vi "Configurator_Main.vi"() -> ()   [LabVIEW 2013]
doc: "This is the main VI for the configuration editor."
uses:
  Controls/StateCluster.ctl
  vi.lib/CEF_TreeControl/Repository/NISE_CEF_Repository.lvclass
  vi.lib/CEF_TreeControl/Node/NodeRef.ctl
  vi.lib/CEF_TreeControl/Node/NISE_CEF_Node.lvclass
  vi.lib/CEF_TreeControl/Node/UserEventRef.ctl
  vi.lib/CEF_TreeControl/Controls/EventCluster.ctl
  Controls/AddMessage.ctl
  Controls/MoveMessage.ctl
  Classes/cRIO/cRIO.lvclass
  Classes/cRIO Repo/cRIORepo.lvclass
  <vilib>/NI/AMC/Read Termination Message.vi
  <vilib>/NI/AMC/Create Single Message.vi
  <vilib>/NI/AMC/Update Message Routing Info.vi
  <vilib>/NI/AMC/Send Message.vi
  <vilib>/NI/AMC/Globals.vi
  <vilib>/NI/AMC/AMC.lvlib
  vi.lib/CEF_TreeControl/NISE_CEF_TreeControl.lvlib
panel:
  in  "View":string(tree)
  in  "Exit":bool
  # "Configurator"
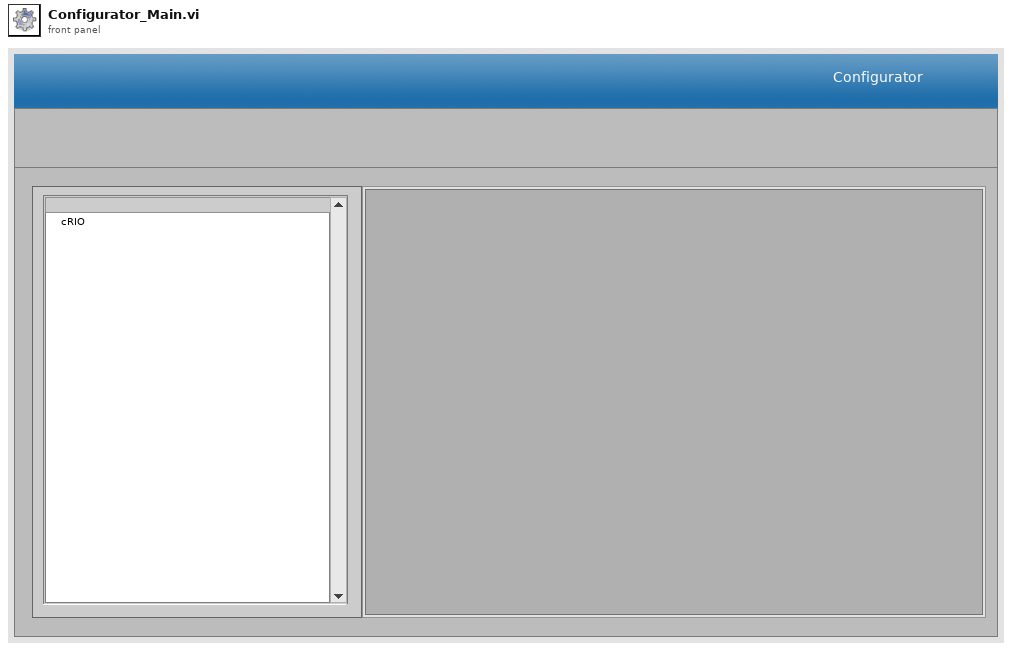
[diagram p1: front panel]
types:
  T1 = typedef "StateCluster.ctl" = cluster{"repository":refnum<class "NISE_CEF_Repository.lvclass">, "root":T2, "unsaved changes":bool, "current path":path, "user event ref":T3, "glyph path":path, "classes path":path}
  T2 = typedef "NISE_CEF_Node.lvclass/NodeRef.ctl" = refnum<data-value>
  T3 = typedef "NISE_CEF_Node.lvclass/UserEventRef.ctl" = refnum<user-event>
  T4 = typedef "AMC.lvlib/Message Queue.ctl" = refnum<queue>
  T5 = typedef "AddMessage.ctl" = cluster{"node type":string, "to add to":string}
  T6 = typedef "MoveMessage.ctl" = cluster{"node ref":T2, "new parent":T2}
  T7 = typedef "NISE_CEF_TreeControl.lvlib/EventCluster.ctl" = cluster{"command":string, "data":string}
  T8 = typedef "FilePaths.ctl" = cluster{"glyphs":path, "classes":path}
  T9 = typedef "NISE_CEF_Node.lvclass/Summary.ctl" = cluster{"ID":string, "parent ID":string, "node type":string, "text":string, "additional text":string, "glyph":string, "depth":i32}
  T10 = typedef "LVPoint32TypeDef.ctl" = cluster{"Horizontal":i32, "Vertical":i32}
  T11 = cluster{"data name":string, "drag data":variant}[]
  T12 = typedef "NISE_CEF_Node.lvclass/NodeMenuOptions.ctl" = cluster{"removable":bool, "movable":bool, "duplicate":bool}
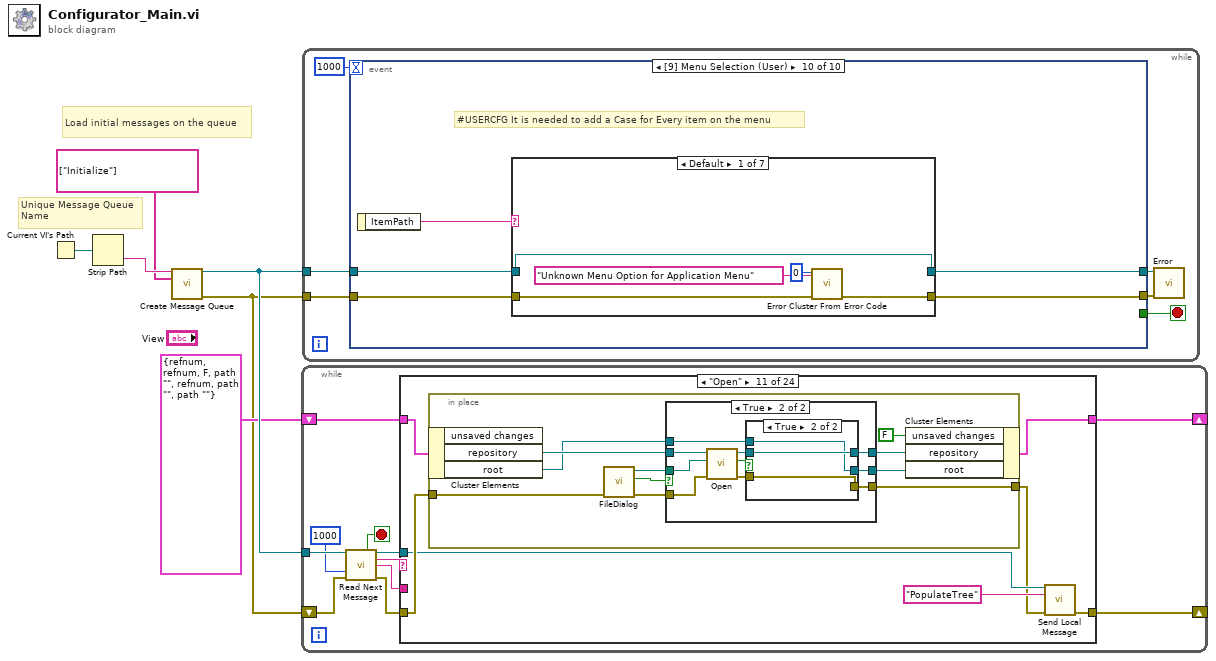
[diagram p0: block diagram]
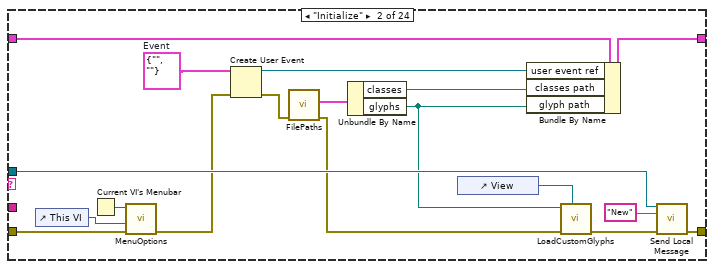
[diagram p3: hidden frame]
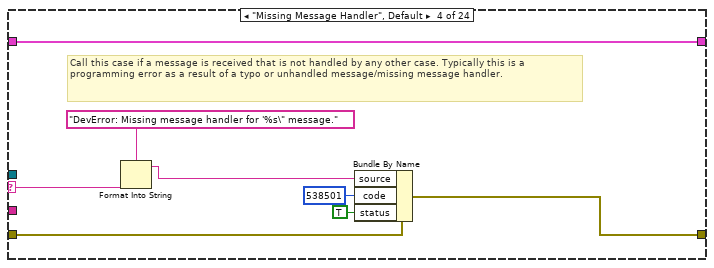
[diagram p5: hidden frame]
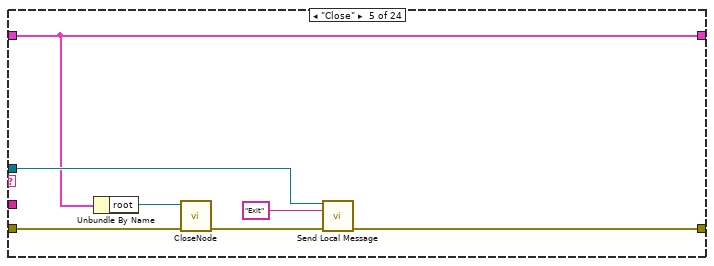
[diagram p6: hidden frame]
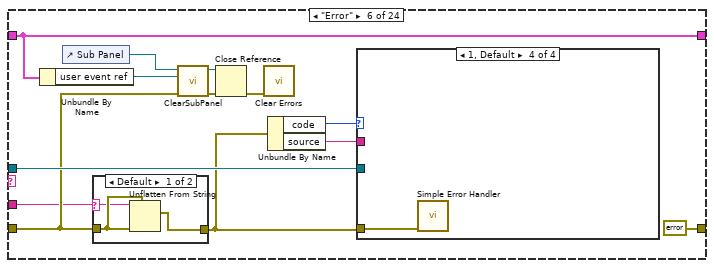
[diagram p7: hidden frame]
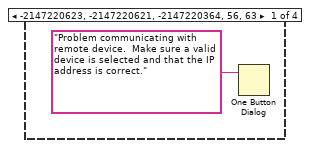
[diagram p9: hidden frame]
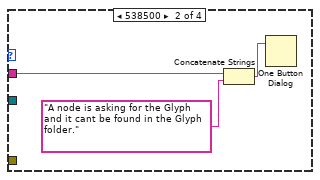
[diagram p10: hidden frame]
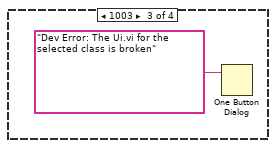
[diagram p11: hidden frame]
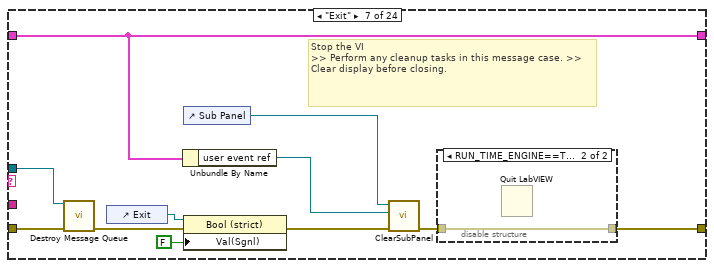
[diagram p12: hidden frame]
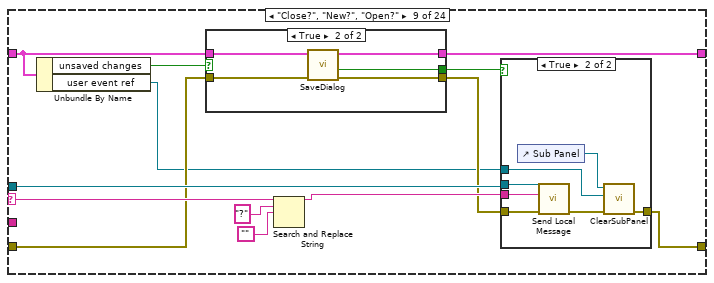
[diagram p15: hidden frame]
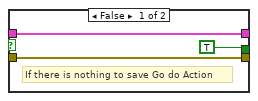
[diagram p16: hidden frame]
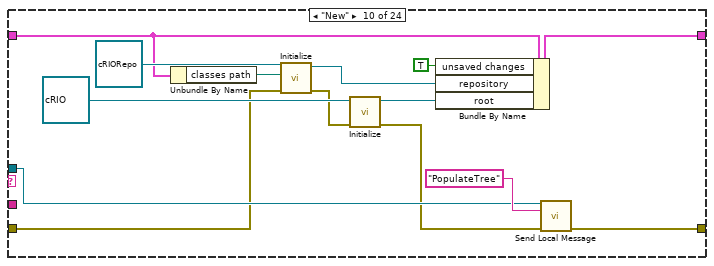
[diagram p18: hidden frame]
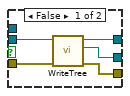
[diagram p20: hidden frame]
diagram:
  # "Unique Message Queue Name"
  # "Load initial messages on the queue"
  n1 = Current VI's Path() -> (path=w5:path)
  n2 = Strip Path(path=w5) -> (name=w6:string)  [unwired: 1 out]
  n3 = call <vilib>:"Create Message Queue.vi"("message queue name"=w6, "initial message names"=string[] ["Initialize"]) -> ("message queue out"=w3:T4, "error out"=w1:errorcluster)  [unwired: 12 in]
  n4 = while "Message Processor" {
    shift-right: [w13] -> _
    shift-left: w1 -> [w12]
    tunnel: w3 -> [w11]
    shift-right: [w9] -> _
    shift-left: T1 {"repository"=refnum, "root"=refnum, "unsaved changes"=FALSE, "current path"=path "", "user event ref"=refnum, "glyph path"=path "", "classes path"=path ""} -> [w8]
    stop <- w17 stop-if-true
    n5 = call <vilib>:"Read Next Message.vi"("message queue in"=w11, "timeout (1 ms)"=1000, "error in"=w12) -> ("exit process?"=w17:bool, "message queue out"=w7:T4, "message name"=w16:string, "message value"=w15:string, "error out"=w14:errorcluster)  [unwired: 5 in, 3 out]
    n6 = case shown="\"Open\"" w16 {
      selector: w16 -> [_ _ _ w46 _ _ _ _ w101 _ _ _ _ _ _ _ _ w277 _ _ _ _ _ _]
      tunnel: w15 -> [_ _ _ _ _ w56 _ _ _ _ _ _ _ w210 _ w247 w258 w275 w311 w332 _ _ w368 w388]
      tunnel: w14 -> [w19 w37 w39 w44 w49 w59 w88 w92 w94 w122 w140 w176 w202 w217 w230 w236 w257 w280 w313 w331 w348 w358 w367 w386]
      tunnel: [w19 w31 w39 w43 w53 errorcluster {"status"=FALSE, "code"=0, "source"=""} ("error out") w80 w92 w105 w134 w136 w180 w204 w214 w230 w239 w261 w283 w317 w328 w342 w353 w364 w381] -> w13
      tunnel: [w18 w26 w38 w45 w51 w64 w79 w91 w96 w132 w141 w183 w203 w211 w229 w233 w262 w284 w315 w333 w352 w357 w362 w389] -> w9
      tunnel: w8 -> [w18 w27 w38 w45 w51 w64 w79 w91 w97 w126 w142 w178 w201 w212 w229 w234 w262 w284 w316 w333 w352 w357 w362 w389]
      tunnel: w7 -> [_ w30 _ _ w52 w67 w87 _ w104 w133 w138 w179 _ w213 _ _ _ w278 _ _ _ _ w363 w380]
      frame "------------Generic Operations------------" {
        # "Dummy case to add a seperation in the Case Structure menu"
      }
      frame "Initialize" {
        w21 = T7 {"command"="", "data"=""}  # Event
        n7 = control-ref of="This VI"() -> (w36:refnum<vi>)
        n8 = Current VI's Menubar() -> (w35:refnum<k9>)
        n9 = call "MenuOptions.vi"("error in"=w37, "VI ref"=w36, "menu ref in"=w35) -> ("error out"=w25:errorcluster)  [unwired: 7 in, 1 out]
        n10 = Create User Event(user event datatype=w21, error in=w25) -> (user event=w20:refnum<user-event>, error out=w24:errorcluster)
        n11 = call "FilePaths.vi"("error in"=w24) -> ("error out"=w29:errorcluster, "paths"=w28:T8)  [unwired: 9 in]
        n12 = Unbundle By Name(w28) -> ("classes"=w23:path, "glyphs"=w22:path)
        n13 = control-ref of="View"() -> (w34:refnum<vi>)
        n14 = Bundle By Name(cluster=w27, "user event ref"=w20, "classes path"=w23, "glyph path"=w22) -> (w26:T1)
        n15 = call "LoadCustomGlyphs.vi"("tree ref"=w34, "error in"=w29, "glyph directory"=w22) -> ("error out"=w32:errorcluster)  [unwired: 8 in]
        n16 = call <vilib>:"Send Local Message.vi"("message queue in"=w30, "message name"="New" ("Message Name"), "error in"=w32) -> ("error out"=w31:errorcluster)  [unwired: 10 in, 2 out]
      }
      frame "", "Idle" {
      }
      frame "Missing Message Handler", Default {
        # "Call this case if a message is received that is not handled by any other case. Typically this is a programming error as a result of a typo or unhandled message/missing message handler."
        n17 = Format Into String(format string="DevError: Missing message handler for '%s\" message." ("message"), w46) -> (resulting string=w40:string)  [unwired: 2 in, 1 out]
        n18 = Bundle By Name(cluster=w44, "source"=w40, "code"=538501, "status"=TRUE) -> (w43:errorcluster)
      }
      frame "Close" {
        n19 = Unbundle By Name(w51) -> ("root"=w50:T2)
        n20 = call "CloseNode.vi"("error in"=w49, "node ref"=w50) -> ("error out"=w48:errorcluster)  [unwired: 9 in]
        n21 = call <vilib>:"Send Local Message.vi"("message queue in"=w52, "message name"="Exit", "error in"=w48) -> ("error out"=w53:errorcluster)  [unwired: 10 in, 2 out]
      }
      frame "Error" {
        n22 = Unbundle By Name(w64) -> ("user event ref"=w62:T3)
        n23 = control-ref of="Sub Panel"() -> (w63:refnum<vi>)
        n24 = case shown="Default" w56 {
          selector: w56 -> [w69 _]
          tunnel: w59 -> [w70 w71]
          tunnel: [w68 w71] -> w58
          frame Default {
            n25 = Unflatten From String(type=w70, binary string=w69, error in (no error)=w70) -> (value=w68:errorcluster)  [unwired: 2 in, 2 out]
          }
          frame "" {
          }
        }
        n26 = call "ClearSubPanel.vi"("error in"=w59, "user event ref"=w62, "sub panel ref in"=w63) -> ("error out"=w61:errorcluster, "sub panel ref out"=w60:refnum<vi>)  [unwired: 7 in]
        n27 = Close Reference(reference=w60, error in (no error)=w61) -> (error out=w57:errorcluster)
        n28 = call <vilib>:"Clear Errors.vi"("error in (no error)"=w57) -> ()  [unwired: 6 in, 1 out]
        n29 = Unbundle By Name(w58) -> ("code"=w65:i32, "source"=w55:string)
        n30 = case shown="1, Default" w65 {
          tunnel: w67 -> [_ _ _ _]
          tunnel: w58 -> [_ _ _ w77]
          tunnel: w55 -> [_ w75 _ _]
          frame -2147220623, -2147220621, -2147220364, 56, 63 {
            n31 = One Button Dialog(message="Problem communicating with remote device.  Make sure a valid device is selected and that the IP address is correct.") -> ()  [unwired: 1 in, 1 out]
          }
          frame 538500 {
            n32 = Concatenate Strings(w75, "A node is asking for the Glyph and it cant be found in the Glyph folder." ("message")) -> (w73:string)
            n33 = One Button Dialog(message=w73) -> ()  [unwired: 1 in, 1 out]
          }
          frame 1003 {
            n34 = One Button Dialog(message="Dev Error: The Ui.vi for the selected class is broken") -> ()  [unwired: 1 in, 1 out]
          }
          frame 1, Default {
            n35 = call <vilib>:"Simple Error Handler.vi"("error in (no error)"=w77) -> ()  [unwired: 1 in, 8 out]
          }
        }
      }
      frame "Exit" {
        # "Stop the VI                                                                             >> Perform any cleanup tasks in this message case. >> Clear display before closing."
        n36 = call <vilib>:"Destroy Message Queue.vi"("message queue in"=w87, "error in"=w88) -> ("error out"=w84:errorcluster)  [unwired: 11 in, 2 out]
        n37 = control-ref of="Exit"() -> (w86:refnum<vi>)
        n38 = Unbundle By Name(w79) -> ("user event ref"=w78:T3)
        n39 = control-ref of="Sub Panel"() -> (w83:refnum<vi>)
        n40 = property class="Bool (strict)"(reference=w86, error in=w84, "Val(Sgnl)"=FALSE ("Exit")) -> (error out=w82:errorcluster)  [unwired: 1 out]
        n41 = call "ClearSubPanel.vi"("error in"=w82, "user event ref"=w78, "sub panel ref in"=w83) -> ("error out"=w81:errorcluster)  [unwired: 7 in, 1 out]
        n42 = disable-structure shown="RUN_TIME_ENGINE==True" {
          disable-tunnel: [w89 w90] -> w80
          disable-tunnel: w81 -> [w89 w90]
          frame condition #0 (active) {
          }
          frame condition #1 {
            n43 = Quit LabVIEW() -> ()  [unwired: 1 in]
          }
        }
      }
      frame "------------Menu Operations--------------" {
        # "Dummy case to add a seperation in the Case Structure menu"
      }
      frame "Close?", "New?", "Open?" {
        n44 = Unbundle By Name(w97) -> ("unsaved changes"=w99:bool, "user event ref"=w93:T3)
        n45 = case shown="True" w99 {
          tunnel: [TRUE ("SaveFlag") w113] -> w98
          tunnel: w97 -> [w107 w112]
          tunnel: [w107 w111] -> w96
          tunnel: w94 -> [w106 w110]
          tunnel: [w106 w109] -> w95
          frame False {
            # "If there is nothing to save Go do Action"
          }
          frame True {
            n46 = call "SaveDialog.vi"("error in"=w110, "state in"=w112) -> ("error out"=w109:errorcluster, "new"=w113:bool, "state out"=w111:T1)  [unwired: 7 in]
          }
        }
        n47 = Search and Replace String(input string=w101, search string="?", replace string="") -> (result string=w100:string)  [unwired: 5 in, 3 out]
        n48 = case shown="True" w98 {
          tunnel: w95 -> [w114 w121]
          tunnel: [w114 w117] -> w105
          tunnel: w104 -> [_ w120]
          tunnel: w100 -> [_ w119]
          tunnel: w93 -> [_ w116]
          frame False {
          }
          frame True {
            n49 = control-ref of="Sub Panel"() -> (w115:refnum<vi>)
            n50 = call <vilib>:"Send Local Message.vi"("message queue in"=w120, "message name"=w119, "error in"=w121) -> ("error out"=w118:errorcluster)  [unwired: 10 in, 2 out]
            n51 = call "ClearSubPanel.vi"("error in"=w118, "user event ref"=w116, "sub panel ref in"=w115) -> ("error out"=w117:errorcluster)  [unwired: 7 in, 1 out]
          }
        }
      }
      frame "New" {
        n52 = Unbundle By Name(w126) -> ("classes path"=w125:path)
        n53 = call-dynamic "Initialize.vi"("error in"=w122, "path"=w125, "repository in"=refnum<class "cRIORepo.lvclass"> refnum ("cRIORepo.lvclass")) -> ("error out"=w124:errorcluster, "repository out"=w127:refnum<class "cRIORepo.lvclass">)  [unwired: 7 in]
        n54 = call-dynamic "Initialize.vi"("error in"=w124, "cRIO in"=refnum<class "cRIO.lvclass"> refnum ("cRIO.lvclass")) -> ("error out"=w123:errorcluster, "data value reference"=w129:T2)  [unwired: 7 in, 1 out]
        n55 = Bundle By Name(cluster=w126, "unsaved changes"=TRUE ("SaveFlag"), "repository"=w127, "root"=w129) -> (w132:T1)
        n56 = call <vilib>:"Send Local Message.vi"("message queue in"=w133, "message name"="PopulateTree", "error in"=w123) -> ("error out"=w134:errorcluster)  [unwired: 10 in, 2 out]
      }
      frame "Open" {
        n57 = in-place {
          in-place-border: w140 -> [w143]
          in-place-border: [w149] -> w137
          n58 = in-place-cluster #1(w142) -> ("repository"=w152:refnum<class "NISE_CEF_Repository.lvclass">, "root"=w147:T2)  [unwired: 1 out]
          n59 = call "FileDialog.vi"("error in"=w143) -> ("error out"=w144:errorcluster, "Valid"=w146:bool, "selected path"=w145:path)  [unwired: 7 in, 1 out]
          n60 = case shown="True" w146 {
            tunnel: w152 -> [w153 w165]
            tunnel: [w153 w163] -> w150
            tunnel: [w154 w161] -> w149
            tunnel: [w155 w160] -> w148
            tunnel: w145 -> [_ w158]
            tunnel: w144 -> [w154 w157]
            tunnel: w147 -> [w155 w156]
            frame False {
            }
            frame True {
              n61 = call-dynamic "Open.vi"("error in"=w157, "file path"=w158, "repository in"=w165) -> ("error out"=w162:errorcluster, "invalid?"=w159:bool, "repository out"=w164:refnum<class "NISE_CEF_Repository.lvclass">)  [unwired: 6 in]
              n62 = case shown="True" w159 {
                tunnel: w164 -> [w170 w173]
                tunnel: [w169 w173] -> w163
                tunnel: w162 -> [w168 w172]
                tunnel: [w167 w172] -> w161
                tunnel: [w166 w171] -> w160
                tunnel: w156 -> [_ w171]
                frame False {
                  n63 = call-dynamic "WriteTree.vi"("error in"=w168, "repository in"=w170) -> ("error out"=w167:errorcluster, "root"=w166:T2, "repository out"=w169:refnum<class "NISE_CEF_Repository.lvclass">)  [unwired: 7 in]
                }
                frame True {
                }
              }
            }
          }
          n64 = in-place-cluster #1("unsaved changes"=FALSE ("SaveFlag"), "repository"=w150, "root"=w148) -> (w141:T1)
        }
        n65 = call <vilib>:"Send Local Message.vi"("message queue in"=w138, "message name"="PopulateTree", "error in"=w137) -> ("error out"=w136:errorcluster)  [unwired: 10 in, 2 out]
      }
      frame "Save" {
        n66 = in-place {
          in-place-border: w176 -> [w187]
          in-place-border: [w186] -> w175
          in-place-border: [w184] -> w174
          n67 = in-place-cluster #2(w178) -> ("current path"=w185:path, "root"=w188:T2, "repository"=w190:refnum<class "NISE_CEF_Repository.lvclass">)
          n68 = Empty String/Path?(string/path=w185) -> (empty?=w184:bool)
          n69 = call-dynamic "ReadTree.vi"("error in"=w187, "root"=w188, "repository in"=w190) -> ("error out"=w186:errorcluster, "repository out"=w189:refnum<class "NISE_CEF_Repository.lvclass">)  [unwired: 7 in]
          n70 = in-place-cluster #2("current path"=w185, "root"=w188, "repository"=w189) -> (w177:T1)
        }
        n71 = case shown="True" w174 {
          tunnel: w177 -> [w194 w196]
          tunnel: [w193 w195] -> w183
          tunnel: [w192 w197] -> w181
          tunnel: w175 -> [w191 w198]
          frame False {
            n72 = call "Save.vi"("error in"=w191, "state in"=w194) -> ("error out"=w192:errorcluster, "state out"=w193:T1)  [unwired: 8 in]
          }
          frame True {
            # "Empty path use Dialog"
            n73 = call "SaveAs.vi"("error in"=w198, "state in"=w196) -> ("error out"=w197:errorcluster, "state out"=w195:T1)  [unwired: 7 in, 1 out]
          }
        }
        n74 = call <vilib>:"Send Local Message.vi"("message queue in"=w179, "message name"="PopulateTree", "error in"=w181) -> ("error out"=w180:errorcluster)  [unwired: 10 in, 2 out]
      }
      frame "SaveAs" {
        n75 = in-place {
          in-place-border: w202 -> [w206]
          in-place-border: [w205] -> w200
          n76 = in-place-cluster #3(w201) -> ("root"=w207:T2, "repository"=w209:refnum<class "NISE_CEF_Repository.lvclass">)
          n77 = call-dynamic "ReadTree.vi"("error in"=w206, "root"=w207, "repository in"=w209) -> ("error out"=w205:errorcluster, "repository out"=w208:refnum<class "NISE_CEF_Repository.lvclass">)  [unwired: 7 in]
          n78 = in-place-cluster #3("root"=w207, "repository"=w208) -> (w199:T1)
        }
        n79 = call "SaveAs.vi"("error in"=w200, "state in"=w199) -> ("error out"=w204:errorcluster, "state out"=w203:T1)  [unwired: 7 in, 1 out]
      }
      frame "Custom View" {
        n80 = in-place {
          in-place-border: w217 -> [w228]
          in-place-border: [w227] -> w215
          in-place-border: w210 -> [w218]
          n81 = in-place-cluster #4(w212) -> ("repository"=w222:refnum<class "NISE_CEF_Repository.lvclass">, "root"=w221:T2)
          n82 = call-dynamic "ReadTree.vi"("error in"=w228, "root"=w221, "repository in"=w222) -> ("error out"=w225:errorcluster, "repository out"=w224:refnum<class "NISE_CEF_Repository.lvclass">)  [unwired: 7 in]
          n83 = call-dynamic "CustomView.vi"("error in"=w225, "view name"=w218, "repository in"=w224) -> ("error out"=w226:errorcluster, "repository out"=w223:refnum<class "NISE_CEF_Repository.lvclass">)  [unwired: 7 in]
          n84 = call-dynamic "WriteTree.vi"("error in"=w226, "repository in"=w223) -> ("error out"=w227:errorcluster, "root"=w219:T2, "repository out"=w220:refnum<class "NISE_CEF_Repository.lvclass">)  [unwired: 7 in]
          n85 = in-place-cluster #4("repository"=w220, "root"=w219) -> (w211:T1)
        }
        n86 = call <vilib>:"Send Local Message.vi"("message queue in"=w213, "message name"="PopulateTree", "error in"=w215) -> ("error out"=w214:errorcluster)  [unwired: 10 in, 2 out]
      }
      frame "-------TreeControl Operations-----------" {
        # "Dummy case to add a seperation in the Case Structure menu"
      }
      frame "AddNode" {
        n87 = Unflatten From String(type=T5 {"node type"="", "to add to"=""} ("input cluster"), binary string=w247) -> (value=w245:T5)  [unwired: 3 in, 2 out]
        n88 = Unbundle By Name(w245) -> ("to add to"=w242:string, "node type"=w232:string)
        n89 = in-place {
          in-place-border: w236 -> [w253]
          in-place-border: [w252] -> w235
          in-place-border: w232 -> [w251]
          in-place-border: [w250] -> w231
          n90 = in-place-cluster #5(w234) -> ("repository"=w255:refnum<class "NISE_CEF_Repository.lvclass">)
          n91 = call-dynamic "GetClassPath.vi"("error in"=w253, "class name"=w251, "Repository in"=w255) -> ("error out"=w252:errorcluster, "class path"=w250:path, "Repository out"=w254:refnum<class "NISE_CEF_Repository.lvclass">)  [unwired: 6 in]
          n92 = in-place-cluster #5("repository"=w254) -> (w233:T1)
        }
        n93 = control-ref of="View"() -> (w237:refnum<vi>)
        n94 = call <vilib>:"Get LV Class Default Value.vi"("error in (no error)"=w235, "class path"=w231) -> ("error out"=w248:errorcluster, "object"=w249:refnum<class>)  [unwired: 8 in]
        n95 = To More Specific Class(target class=refnum<class "NISE_CEF_Node.lvclass"> refnum ("Node.lvclass"), reference=w249, error in=w248) -> (specific class reference=w244:refnum<class "NISE_CEF_Node.lvclass">, error out=w241:errorcluster)
        n96 = call "AddNode.vi"("error in"=w241, "node in"=w244, "parent node ID"=w242) -> ("error out"=w240:errorcluster, "summary"=w238:T9[])  [unwired: 7 in]
        n97 = call "PopulateTreeSumary.vi"("error in"=w240, "array"=w238, "tree ref in"=w237) -> ("error out"=w239:errorcluster)  [unwired: 8 in]
      }
      frame "Duplicate" {
        n98 = call "IDtoNode.vi"("error in"=w257, "ID"=w258) -> ("error out"=w259:errorcluster, "invalid Id"=w256:bool, "node ref"=w260:T2)  [unwired: 7 in]
        n99 = case shown="False" w256 {
          tunnel: [w271 w272] -> w261
          tunnel: w260 -> [w269 _]
          tunnel: w259 -> [w266 w272]
          frame False {
            n100 = call "DuplicateNode.vi"("same parent?"=TRUE ("s"), "error in"=w266, "node ref in"=w269) -> ("error out"=w267:errorcluster, "new node ref"=w268:T2)  [unwired: 7 in]
            n101 = call "Summary.vi"("error in"=w267, "node self ref"=w268) -> ("error out"=w264:errorcluster, "summary"=w263:T9[])  [unwired: 8 in]
            n102 = control-ref of="View"() -> (w270:refnum<vi>)
            n103 = call "PopulateTreeSumary.vi"("error in"=w264, "array"=w263, "tree ref in"=w270) -> ("error out"=w271:errorcluster)  [unwired: 8 in]
          }
          frame True {
          }
        }
      }
      frame "CustomMenuAction" {
        n104 = Match Pattern(string=w275, regular expression=":") -> (before substring=w274:string, after substring=w273:string)  [unwired: 1 in, 2 out]
        n105 = call "IDtoNode.vi"("error in"=w280, "ID"=w273) -> ("error out"=w281:errorcluster, "invalid Id"=w279:bool, "node ref"=w282:T2)  [unwired: 7 in]
        n106 = case shown="False" w279 {
          tunnel: [w285 w308] -> w283
          tunnel: w282 -> [w292 _]
          tunnel: w281 -> [w289 w308]
          tunnel: w278 -> [w291 _]
          tunnel: w277 -> [_ _]
          tunnel: w274 -> [w287 _]
          frame False {
            n107 = control-ref of="View"() -> (w290:refnum<vi>)
            n108 = in-place {
              in-place-border: w291 -> [w306]
              in-place-border: w290 -> [w304]
              in-place-border: w289 -> [w303]
              in-place-border: [w302] -> w286
              in-place-border: [w301] -> w288
              in-place-border: w287 -> [w300]
              n109 = in-place-dvr #6(w292) -> (w307:refnum<class "NISE_CEF_Node.lvclass">)  [unwired: 1 out]
              n110 = call-dynamic "MenuHandler.vi"("tree control"=w304, "message queue out"=w306, "error in (no error)"=w303, "menu string"=w300, "NISE_CEF_Node in"=w307) -> ("error out"=w302:errorcluster, "Unhandled"=w301:bool, "NISE_CEF_Node out"=w305:refnum<class "NISE_CEF_Node.lvclass">)  [unwired: 4 in]
              n111 = in-place-dvr #6(w305) -> ()  [unwired: 2 out]
            }
            n112 = case shown="True" w288 {
              tunnel: w287 -> [_ w298]
              tunnel: w286 -> [w293 w297]
              tunnel: [w293 w296] -> w285
              frame False {
              }
              frame True {
                # "Generates Error"
                n113 = Concatenate Strings("Unknown Menu item command:  " ("message"), w298) -> (w295:string)
                n114 = call <vilib>:"Error Cluster From Error Code.vi"("error in (no error)"=w297, "error message (\"\")"=w295, "error code (0)"=538502) -> ("error out"=w296:errorcluster)  [unwired: 6 in]
              }
            }
          }
          frame True {
          }
        }
      }
      frame "RefreshNode" {
        # "Refreshes the node in the Tree               Sets the save flag to true                       This case can be called from the UIs of the nodes"
        n115 = call "IDtoNode.vi"("error in"=w313, "ID"=w311) -> ("error out"=w312:errorcluster, "invalid Id"=w309:bool, "node ref"=w310:T2)  [unwired: 7 in]
        n116 = case shown="True" w309 {
          tunnel: [w324 w326] -> w317
          tunnel: w312 -> [w319 w326]
          tunnel: w310 -> [w318 _]
          frame False {
            n117 = call "Summary.vi"("error in"=w319, "node self ref"=w318) -> ("error out"=w321:errorcluster, "summary"=w320:T9[])  [unwired: 8 in]
            n118 = control-ref of="View"() -> (w322:refnum<vi>)
            n119 = call "RefreshSubTree.vi"("error in"=w321, "node information"=w320, "tree ref in"=w322) -> ("error out"=w325:errorcluster, "tree ref out"=w323:refnum<vi>)  [unwired: 7 in]
            n120 = Close Reference(reference=w323, error in (no error)=w325) -> (error out=w324:errorcluster)
          }
          frame True {
          }
        }
        n121 = Bundle By Name(cluster=w316, "unsaved changes"=TRUE ("SaveFlag")) -> (w315:T1)
      }
      frame "RemoveNode" {
        n122 = call "IDtoNode.vi"("error in"=w331, "ID"=w332) -> ("error out"=w330:errorcluster, "invalid Id"=w327:bool, "node ref"=w329:T2)  [unwired: 7 in]
        n123 = case shown="False" w327 {
          tunnel: w330 -> [w339 w340]
          tunnel: w329 -> [w338 _]
          tunnel: [w334 w340] -> w328
          frame False {
            n124 = call "RemoveNode.vi"("error in"=w339, "node"=w338) -> ("error out"=w335:errorcluster, "node ID"=w337:string)  [unwired: 8 in]
            n125 = control-ref of="View"() -> (w336:refnum<vi>)
            n126 = call "ClearTreeNode.vi"("error in"=w335, "tag"=w337, "tree reference"=w336) -> ("error out"=w334:errorcluster)  [unwired: 8 in]
          }
          frame True {
          }
        }
      }
      frame "PopulateTree" {
        n127 = Unbundle By Name(w352) -> ("user event ref"=w341:T3, "root"=w346:T2)
        n128 = call "Summary.vi"("error in"=w348, "depth"=0 ("Depth"), "node self ref"=w346) -> ("error out"=w347:errorcluster, "summary"=w351:T9[])  [unwired: 7 in]
        n129 = control-ref of="This VI"() -> (w349:refnum<vi>)
        n130 = control-ref of="View"() -> (w350:refnum<vi>)
        n131 = call "RefreshEntireTree.vi"("calling VI in"=w349, "error in"=w347, "array"=w351, "tree ref in"=w350) -> ("error out"=w343:errorcluster)  [unwired: 7 in]
        n132 = control-ref of="Sub Panel"() -> (w344:refnum<vi>)
        n133 = call "ClearSubPanel.vi"("error in"=w343, "user event ref"=w341, "sub panel ref in"=w344) -> ("error out"=w342:errorcluster)  [unwired: 7 in, 1 out]
      }
      frame "CleansubPanel" {
        n134 = Unbundle By Name(w357) -> ("user event ref"=w356:T3)
        n135 = control-ref of="Sub Panel"() -> (w359:refnum<vi>)
        n136 = call "ClearSubPanel.vi"("error in"=w358, "user event ref"=w356, "sub panel ref in"=w359) -> ("error out"=w355:errorcluster, "sub panel ref out"=w354:refnum<vi>)  [unwired: 7 in]
        n137 = Close Reference(reference=w354, error in (no error)=w355) -> (error out=w353:errorcluster)
      }
      frame "ActivateNode" {
        n138 = Unbundle By Name(w362) -> ("user event ref"=w361:T3)
        n139 = call "IDtoNode.vi"("error in"=w367, "ID"=w368) -> ("error out"=w360:errorcluster, "invalid Id"=w366:bool, "node ref"=w365:T2)  [unwired: 7 in]
        n140 = case shown="False" w366 {
          tunnel: w365 -> [w375 _]
          tunnel: [w376 w377] -> w364
          tunnel: w360 -> [w373 w377]
          tunnel: w363 -> [w370 _]
          tunnel: w361 -> [w371 _]
          frame False {
            n141 = control-ref of="Sub Panel"() -> (w372:refnum<vi>)
            n142 = call "ClearSubPanel.vi"("error in"=w373, "user event ref"=w371, "sub panel ref in"=w372) -> ("error out"=w374:errorcluster, "sub panel ref out"=w369:refnum<vi>)  [unwired: 7 in]
            n143 = call "LoadNodeUI.vi"("user event out"=w371, "error in"=w374, "sub panel ref in"=w369, "main queue"=w370, "node"=w375) -> ("error out"=w376:errorcluster)  [unwired: 6 in]
          }
          frame True {
          }
        }
      }
      frame "Move" {
        n144 = Unflatten From String(type=T6 {"node ref"=refnum, "new parent"=refnum} ("Cluster"), binary string=w388, error in (no error)=w386) -> (value=w385:T6, error out=w384:errorcluster)  [unwired: 2 in, 1 out]
        n145 = Unbundle By Name(w385) -> ("node ref"=w379:T2, "new parent"=w378:T2)
        n146 = call "MoveNode.vi"("error in"=w384, "new parent"=w378, "node"=w379) -> ("error out"=w382:errorcluster)  [unwired: 8 in]
        n147 = call <vilib>:"Send Local Message.vi"("message queue in"=w380, "message name"="PopulateTree", "error in"=w382) -> ("error out"=w381:errorcluster)  [unwired: 10 in, 2 out]
      }
    }
  }
  n148 = while "User Interface Event Handler" {
    tunnel: w3 -> [w394]
    tunnel: w1 -> [w390]
    stop <- w393 stop-if-true
    n149 = event shown="[9] Menu Selection (User)" {
      selector: _ -> [_ _ _ _ _ _ _ _ _ _]
      dyn-events: _ -> [_ _ _ _ _ _ _ _ _ _]
      timeout: 1000 -> [_ _ _ _ _ _ _ _ _ _]
      tunnel: w394 -> [w397 w405 w429 w481 w509 w516 w545 w549 w559 w564]
      tunnel: [_ _ _ _ TRUE _ _ _ _ _] -> w393
      tunnel: [w397 w405 w426 w479 w505 w516 w542 w549 w557 w563] -> w392
      tunnel: [w396 w401 w425 w478 w506 w512 w541 w546 w555 w561] -> w391
      tunnel: w390 -> [w396 w404 w424 w480 w507 w515 w540 w548 w556 w562]
      event Timeout {
        # "Timeout code can be added here for autosave or Lock Screen"
        n150 = event-data() -> ()  [unwired: 1 in, 1 out]
      }
      event "View": Shortcut Menu Activation? {
        n151 = event-data() -> ("CtlRef"=w411:refnum<vi>, "Coords"=w410:T10, "MenuRef"=w407:refnum<k9>)  [unwired: 1 in]
        n152 = invoke class="Tree (strict)" method="Point To Row Column"(reference=w411, error in=w404, "Point"=w410) -> (error out=w403:errorcluster, "Tag"=w409:string)  [unwired: 5 in, 6 out]
        n153 = call "IDtoNode.vi"("error in"=w403, "ID"=w409) -> ("error out"=w399:errorcluster, "invalid Id"=w406:bool, "node ref"=w408:T2)  [unwired: 7 in]
        n154 = case shown="False" w406 {
          tunnel: w408 -> [w416 _]
          tunnel: w407 -> [w415 _]
          tunnel: [w414 _] -> w402
          tunnel: [w413 _] -> w400
          tunnel: w399 -> [w412 w422]
          tunnel: [w412 w422] -> w398
          frame False {
            n155 = in-place {
              in-place-border: w415 -> [w419]
              in-place-border: [w417] -> w414
              n156 = in-place-dvr #7(w416) -> (w421:refnum<class "NISE_CEF_Node.lvclass">, w418:errorcluster)
              n157 = call-dynamic "ShortcutMenu.vi"("error in"=w418, "menu ref in"=w419, "node in"=w421) -> ("error out"=w417:errorcluster, "node out"=w420:refnum<class "NISE_CEF_Node.lvclass">)  [unwired: 6 in, 1 out]
              n158 = in-place-dvr #7(w420) -> (w413:errorcluster)  [unwired: 1 out]
            }
          }
          frame True {
          }
        }
        n159 = Merge Errors(w400, w402, w398) -> (w401:errorcluster)
        n160 = event-data() -> ()  [unwired: 2 in, 1 out]
      }
      event "View": Shortcut Menu Selection (User) {
        n161 = event-data() -> ("ItemPath"=w428:string, "CtlRef"=w432:refnum<vi>, "Coords"=w433:T10)  [unwired: 1 in]
        n162 = invoke class="Tree (strict)" method="Point To Row Column"(reference=w432, error in=w424, "Point"=w433) -> (error out=w423:errorcluster, "Tag"=w427:string)  [unwired: 5 in, 6 out]
        n163 = Match Pattern(string=w428, regular expression=":") -> (before substring=w431:string, after substring=w430:string)  [unwired: 1 in, 2 out]
        n164 = case shown="Default" w431 {
          selector: w431 -> [w435 _ _ _]
          tunnel: w430 -> [_ _ _ w460]
          tunnel: w429 -> [w442 w449 w455 w462]
          tunnel: w427 -> [w437 w447 w453 w461]
          tunnel: [w439 w446 w452 w458] -> w426
          tunnel: [w440 w445 w450 w456] -> w425
          tunnel: w423 -> [w441 w444 w451 w457]
          frame Default {
            n165 = Concatenate Strings(w435, ":" ("string"), w437) -> (w438:string)
            n166 = call <vilib>:"Send Local Message.vi"("message queue in"=w442, "message name"="CustomMenuAction" ("Message Name"), "message value"=w438, "error in"=w441) -> ("message queue out"=w439:T4, "error out"=w440:errorcluster)  [unwired: 9 in, 1 out]
          }
          frame "Remove" {
            n167 = call <vilib>:"Send Local Message.vi"("message queue in"=w449, "message name"="RemoveNode" ("Message Name"), "message value"=w447, "error in"=w444) -> ("message queue out"=w446:T4, "error out"=w445:errorcluster)  [unwired: 9 in, 1 out]
          }
          frame "Duplicate" {
            n168 = call <vilib>:"Send Local Message.vi"("message queue in"=w455, "message name"="Duplicate" ("Message Name"), "message value"=w453, "error in"=w451) -> ("message queue out"=w452:T4, "error out"=w450:errorcluster)  [unwired: 9 in, 1 out]
          }
          frame "Add" {
            n169 = Bundle By Name(cluster=T5 {"node type"="", "to add to"=""} ("input cluster"), "node type"=w460, "to add to"=w461) -> (w463:T5)
            n170 = Flatten To String(anything=w463) -> (data string=w464:string)  [unwired: 3 in, 2 out]
            n171 = call <vilib>:"Send Local Message.vi"("message queue in"=w462, "message name"="AddNode" ("Message Name"), "message value"=w464, "error in"=w457) -> ("message queue out"=w458:T4, "error out"=w456:errorcluster)  [unwired: 9 in, 1 out]
          }
        }
      }
      event "View": Drop {
        n172 = event-data() -> ("CtlRef"=w484:refnum<vi>, "Coords"=w483:T10)  [unwired: 1 in]
        n173 = invoke class="Tree (strict)" method="Point To Row Column"(reference=w484, error in=w480, "Point"=w483) -> (reference out=w482:refnum<vi>, error out=w477:errorcluster, "Tag"=w474:string)  [unwired: 5 in, 5 out]
        n174 = call "ValidDragDrop.vi"("error in"=w477, "drag over"=w474, "tree ref in"=w482) -> ("error out"=w469:errorcluster, "accepted"=w472:bool, "drag"=w476:string, "tree ref out"=w486:refnum<vi>)  [unwired: 5 in]
        n175 = call "IDtoNode.vi"("error in"=w469, "ID"=w474) -> ("error out"=w470:errorcluster, "invalid Id"=w467:bool, "node ref"=w473:T2)  [unwired: 7 in]
        n176 = call "IDtoNode.vi"("error in"=w470, "ID"=w476) -> ("error out"=w468:errorcluster, "invalid Id"=w466:bool, "node ref"=w475:T2)  [unwired: 7 in]
        n177 = Compound Arithmetic op=AND(w472, invert w467, invert w466) -> (w471:bool)
        n178 = case shown="True" w471 {
          tunnel: w476 -> [_ w502]
          tunnel: w486 -> [_ w504]
          tunnel: [_ TRUE] -> w485
          tunnel: w474 -> [_ w500]
          tunnel: w481 -> [w488 w499]
          tunnel: [w488 w495] -> w479
          tunnel: [w487 w494] -> w478
          tunnel: w475 -> [_ w490]
          tunnel: w473 -> [_ w489]
          tunnel: w468 -> [w487 w491]
          frame False {
          }
          frame True {
            n179 = invoke class="Tree (strict)" method="Edit Tree Items.Move Item"(reference=w504, error in=w491, "tag"=w502, "New Parent"=w500) -> (error out=w492:errorcluster)  [unwired: 3 in, 6 out]
            n180 = Bundle By Name(cluster=T6 {"node ref"=refnum, "new parent"=refnum} ("Cluster"), "new parent"=w489, "node ref"=w490) -> (w498:T6)
            n181 = Flatten To String(anything=w498, error in (no error)=w492) -> (data string=w497:string, error out=w493:errorcluster)  [unwired: 2 in, 1 out]
            n182 = call <vilib>:"Send Local Message.vi"("message queue in"=w499, "message name"="Move", "message value"=w497, "error in"=w493) -> ("message queue out"=w495:T4, "error out"=w494:errorcluster)  [unwired: 9 in, 1 out]
          }
        }
        n183 = event-data("Accepted?"=w485) -> ()  [unwired: 1 in, 1 out]
      }
      event "Exit": Value Change {
        # "Exit the application                                           >> Stop this message generator loop    Cleaning errors if the other loop stop this one"
        n184 = event-data() -> ()  [unwired: 1 in, 1 out]
        n185 = call <vilib>:"Send Local Message.vi"("message queue in"=w509, "message name"="Close", "error in"=w507) -> ("message queue out"=w505:T4, "error out"=w510:errorcluster)  [unwired: 10 in, 1 out]
        n186 = call <vilib>:"Clear Errors.vi"("error in (no error)"=w510) -> ("error out"=w506:errorcluster)  [unwired: 6 in]
      }
      event "View": Drag Starting? {
        n187 = event-data() -> ("Data"=w522:T11, "CtlRef"=w524:refnum<vi>, "Coords"=w523:T10)  [unwired: 1 in]
        n188 = invoke class="Tree (strict)" method="Point To Row Column"(reference=w524, error in=w515, "Point"=w523) -> (error out=w514:errorcluster, "Tag"=w521:string)  [unwired: 5 in, 6 out]
        n189 = call "IDtoNode.vi"("error in"=w514, "ID"=w521) -> ("error out"=w513:errorcluster, "invalid Id"=w520:bool, "node ref"=w519:T2)  [unwired: 7 in]
        n190 = case shown="False" w520 {
          tunnel: w519 -> [w532 _]
          tunnel: [w529 TRUE ("Removable")] -> w517
          tunnel: w513 -> [w528 w538]
          tunnel: [w525 w538] -> w512
          frame False {
            n191 = in-place {
              in-place-border: [w535] -> w531
              in-place-border: w528 -> [w534]
              in-place-border: [w533] -> w527
              n192 = in-place-dvr #8(w532) -> (w537:refnum<class "NISE_CEF_Node.lvclass">)  [unwired: 1 out]
              n193 = call-dynamic "EditOptions.vi"("error in"=w534, "node in"=w537) -> ("error out"=w533:errorcluster, "edit options"=w535:T12, "node out"=w536:refnum<class "NISE_CEF_Node.lvclass">)  [unwired: 6 in, 1 out]
              n194 = in-place-dvr #8(w536) -> (w526:errorcluster)  [unwired: 1 out]
            }
            n195 = Unbundle By Name(w531) -> ("movable"=w530:bool)
            n196 = Merge Errors(w526, w527) -> (w525:errorcluster)
            n197 = Not(x=w530) -> (.not. x?=w529:bool)
          }
          frame True {
          }
        }
        n198 = event-data("Data"=w522, "Drag Mode"=enum32{"copy or move", "copy only", "move only"}."move only", "Discard?"=w517) -> ()  [unwired: 1 in, 1 out]
      }
      event "View": Value Change {
        n199 = event-data() -> ("NewVal"=w543:string)  [unwired: 1 in]
        n200 = call <vilib>:"Send Local Message.vi"("message queue in"=w545, "message name"="ActivateNode" ("Message Name"), "message value"=w543, "error in"=w540) -> ("message queue out"=w542:T4, "error out"=w541:errorcluster)  [unwired: 9 in, 1 out]
      }
      event "View": event type 3.0.xa000003a {
        n201 = event-data() -> ("CtlRef"=w554:refnum<vi>, "Coords"=w551:T10)  [unwired: 1 in]
        n202 = invoke class="Tree (strict)" method="Point To Row Column"(reference=w554, error in=w548, "Point"=w551) -> (reference out=w553:refnum<vi>, error out=w547:errorcluster, "Tag"=w552:string)  [unwired: 5 in, 5 out]
        n203 = call "ValidDragDrop.vi"("error in"=w547, "drag over"=w552, "tree ref in"=w553) -> ("error out"=w546:errorcluster, "accepted"=w550:bool)  [unwired: 5 in, 2 out]
        n204 = event-data("Accepted?"=w550) -> ()  [unwired: 1 in, 1 out]
      }
      event Panel Close? {
        # "Intercepts the upper right close panel operation to allow a smooth shutdown as opposed to immediately killing the app."
        n205 = event-data() -> ()  [unwired: 1 in, 1 out]
        n206 = call <vilib>:"Send Local Message.vi"("message queue in"=w559, "message name"="Close?", "error in"=w556) -> ("message queue out"=w557:T4, "error out"=w555:errorcluster)  [unwired: 10 in, 1 out]
        n207 = event-data("Discard?"=TRUE) -> ()  [unwired: 1 in, 1 out]
      }
      event Menu Selection (User) {
        # "#USERCFG It is needed to add a Case for Every item on the menu"
        n208 = event-data() -> ("ItemPath"=w565:string)  [unwired: 1 in]
        n209 = case shown="Default" w565 {
          tunnel: w564 -> [w570 w575 w580 w585 w590 w595 w604]
          tunnel: [w570 w571 w576 w581 w586 w591 w601] -> w563
          tunnel: w562 -> [w569 w573 w578 w583 w588 w593 w600]
          tunnel: [w568 w572 w577 w582 w587 w592 w598] -> w561
          frame Default {
            n210 = call <vilib>:"Error Cluster From Error Code.vi"("error in (no error)"=w569, "error message (\"\")"="Unknown Menu Option for Application Menu" ("error message (\"\")"), "error code (0)"=0) -> ("error out"=w568:errorcluster)  [unwired: 6 in]
          }
          frame "_File:_New" {
            n211 = call <vilib>:"Send Local Message.vi"("message queue in"=w575, "message name"="New?" ("Message Name"), "error in"=w573) -> ("message queue out"=w571:T4, "error out"=w572:errorcluster)  [unwired: 10 in, 1 out]
          }
          frame "_File:_Open" {
            n212 = call <vilib>:"Send Local Message.vi"("message queue in"=w580, "message name"="Open?" ("Message Name"), "error in"=w578) -> ("message queue out"=w576:T4, "error out"=w577:errorcluster)  [unwired: 10 in, 1 out]
          }
          frame "_File:_Save" {
            n213 = call <vilib>:"Send Local Message.vi"("message queue in"=w585, "message name"="Save" ("Message Name"), "error in"=w583) -> ("message queue out"=w581:T4, "error out"=w582:errorcluster)  [unwired: 10 in, 1 out]
          }
          frame "_File:Save As..." {
            n214 = call <vilib>:"Send Local Message.vi"("message queue in"=w590, "message name"="SaveAs" ("Message Name"), "error in"=w588) -> ("message queue out"=w586:T4, "error out"=w587:errorcluster)  [unwired: 10 in, 1 out]
          }
          frame "_File:_Exit" {
            n215 = call <vilib>:"Send Local Message.vi"("message queue in"=w595, "message name"="Close?" ("Message Name"), "error in"=w593) -> ("message queue out"=w591:T4, "error out"=w592:errorcluster)  [unwired: 10 in, 1 out]
          }
          frame "_Tools:Multiple Parameter Editor" {
            n216 = call <vilib>:"Send Local Message.vi"("message queue in"=w604, "message name"="CleansubPanel", "error in"=w600) -> ("message queue out"=w603:T4, "error out"=w599:errorcluster)  [unwired: 10 in, 1 out]
            n217 = call <vilib>:"Send Local Message.vi"("message queue in"=w603, "message name"="Custom View" ("Message Name"), "message value"="Multiple Variable Editor" ("Message Name"), "error in"=w599) -> ("message queue out"=w601:T4, "error out"=w598:errorcluster)  [unwired: 9 in, 1 out]
          }
        }
      }
    }
    n218 = call "Error.vi"("error in (no error)"=w391, "message queue in"=w392) -> ()  [unwired: 9 in, 1 out]
  }
